vi "Header Entry.vi"(8 "error in (no error)":errorcluster, 10 "Header Data":string, 11 "Byte Stream File in":refnum<file>) -> (0 "error out":errorcluster, 3 "Byte Stream File out":refnum<file>)   [LabVIEW 2018, in "Logging.lvlib"]
uses:
  Logging.lvlib
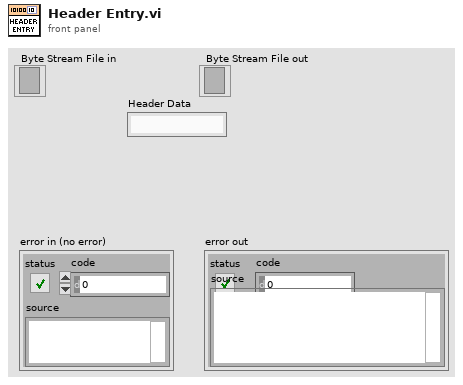
[diagram p1: front panel]
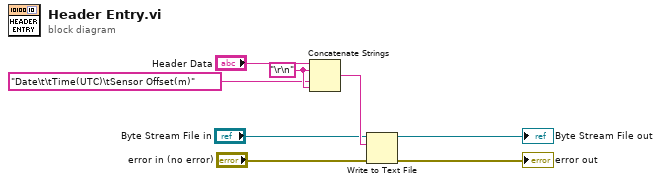
[diagram p0: block diagram]
diagram:
  w2 = "\r\n"
  n1 = Concatenate Strings("Header Data", w2, "Date\t\tTime(UTC)\tSensor Offset(m)" ("string"), w2) -> (w6:string)
  n2 = Write to Text File(file (use dialog)="Byte Stream File in", text=w6, error in="error in (no error)") -> (refnum out=→"Byte Stream File out":refnum<file>, error out=→"error out":errorcluster)  [unwired: 1 in, 1 out]
